vi "tcp_get_devs.vi"(8 "error in":errorcluster, 11 "TCP Network Connection in":refnum<k5>) -> (0 "error out":errorcluster, 2 "devs_info":T1[](array[typedef]), 3 "TCP Network Connection out":refnum<k5>)   [LabVIEW 2021]
uses:
  typedefs/w5500_pck.ctl
  typedefs/w5500_cmd.ctl
  typedefs/dev_full_info.ctl
  typedefs/dev_states.ctl
  typedefs/send_states.ctl
panel:
  out "dev_id":u32
  in  "dev_full_info 2":T1
  in  "devs_number":i32
  in  "w5500_pck":T4
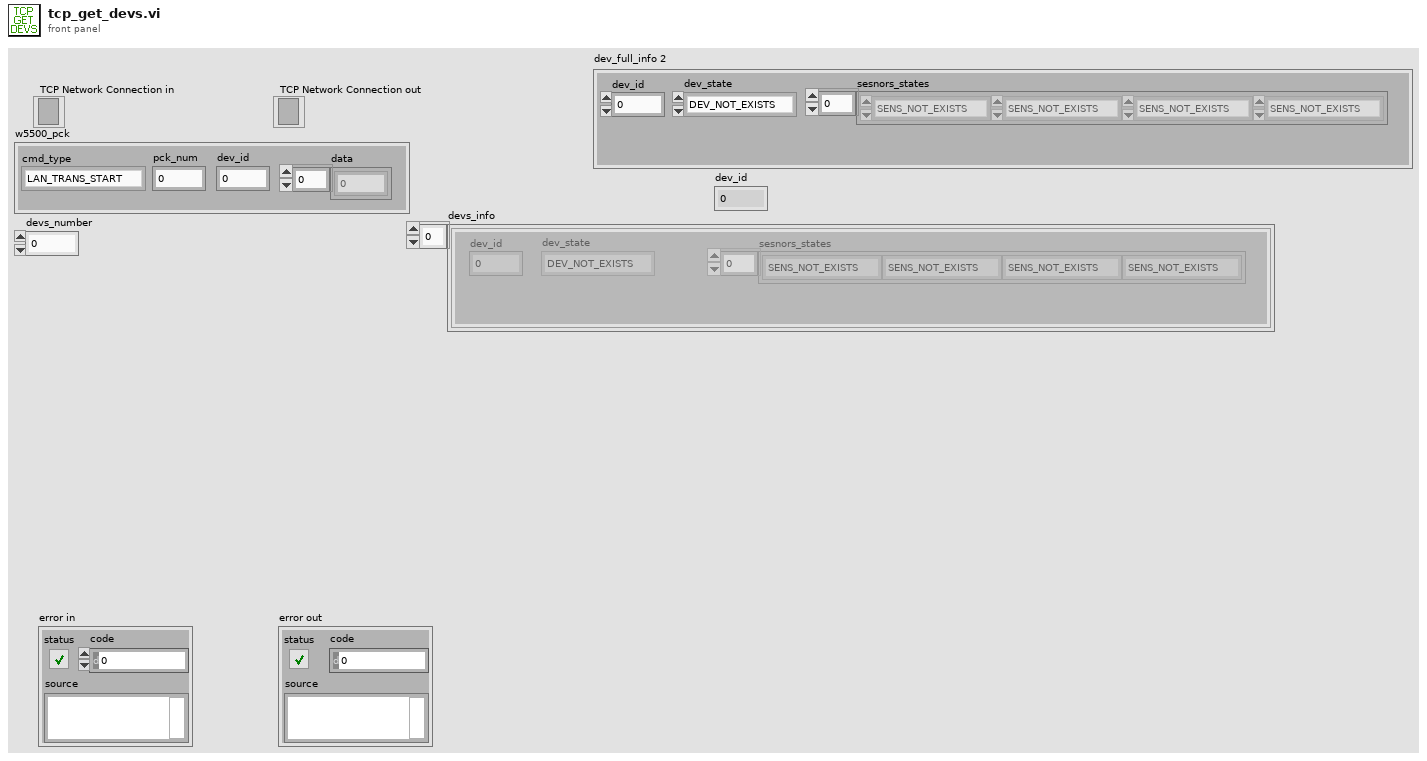
[diagram p1: front panel]
types:
  T1 = typedef "dev_full_info.ctl" = cluster{"dev_id":u32, "dev_state":T2, "sesnors_states":T3[]}
  T2 = typedef "dev_states.ctl" = enum16{"DEV_NOT_EXISTS", "DEV_EXISTS", "DEV_ERROR", "DEV_CRC_ERROR"}
  T3 = typedef "send_states.ctl" = enum16{"SENS_NOT_EXISTS", "SENS_EXISTS"}
  T4 = typedef "w5500_pck.ctl" = cluster{"cmd_type":T5, "pck_num":u32, "dev_id":u32, "data":u8[]}
  T5 = typedef "w5500_cmd.ctl" = enum32{"LAN_TRANS_START", "LAN_DATA_SZ", "LAN_CHUNK_SEND", "LAN_CHUNK_ACK", "LAN_DEVS_INFO", "LAN_DEVS_NUM", "LAN_DEVS_EXS", "LAN_DEVS_ACK", "LAN_CMD_ACK", "LAN_CMD_FIN", "LAN_SND_STAT", "LAN_REQ_STAT", "LAN_ANS_STAT", "LAN_ERR_STAT", "LAN_SETT_SET", "LAN_SETT_GET", "LAN_SETT_ACK", "LAN_SETT_ERR"}
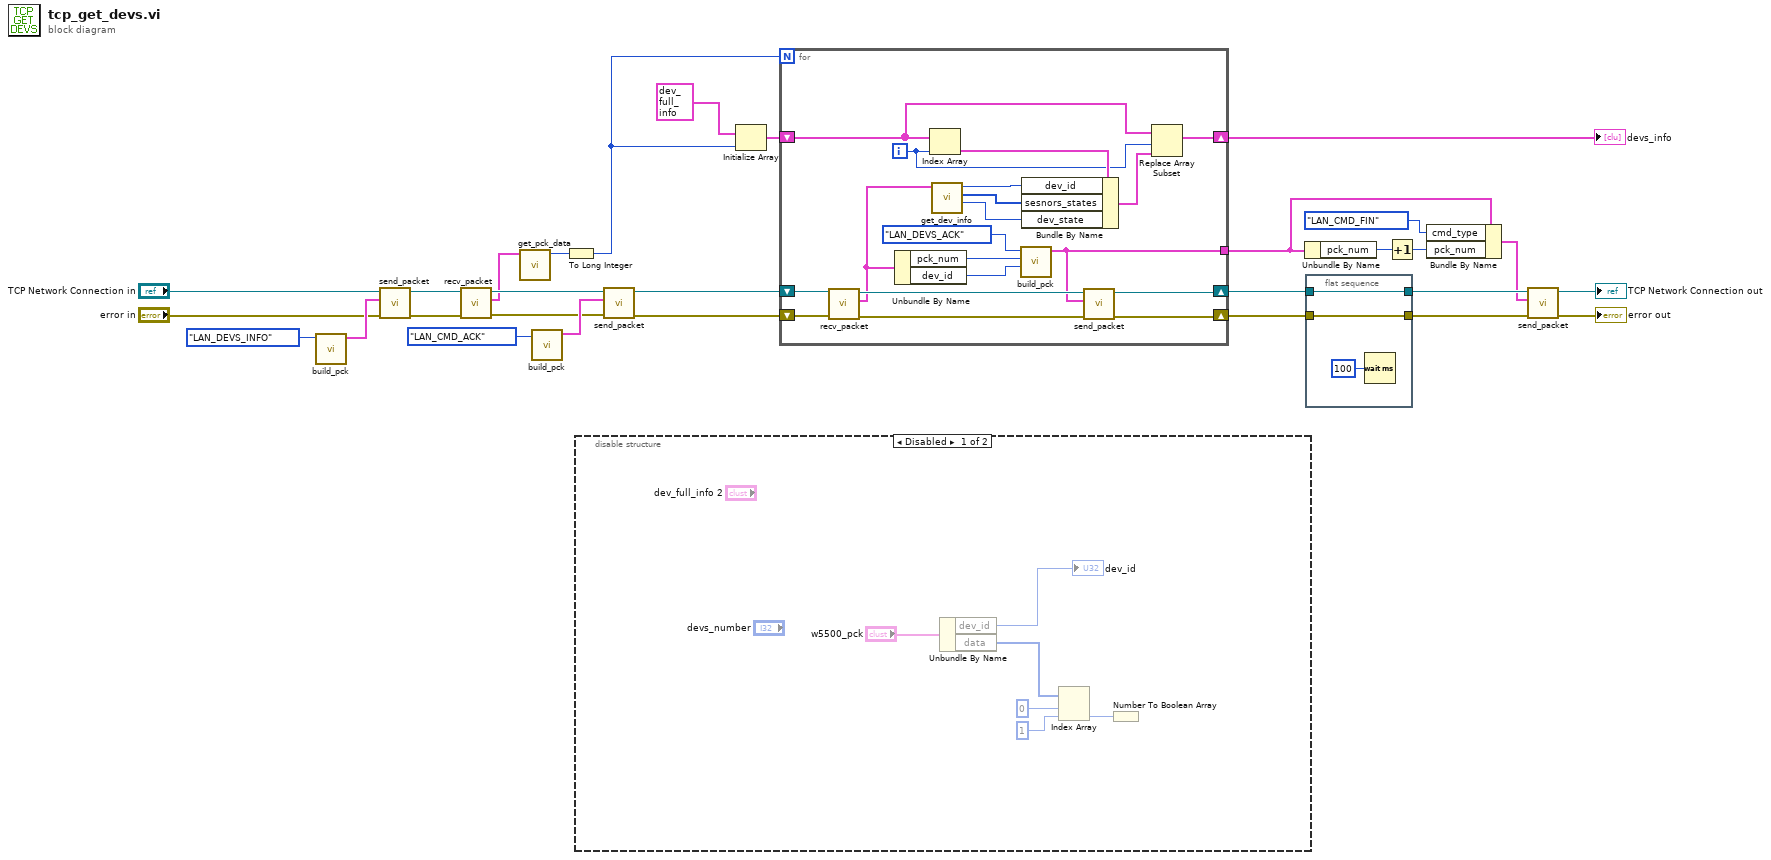
[diagram p0: block diagram]
diagram:
  n1 = call "build_pck.vi"("cmd_type"=w5500_cmd."LAN_DEVS_INFO") -> ("w5500_pck"=w25:T4)  [unwired: 10 in]
  n2 = call "send_packet.vi"("error in (no error)"="error in", "w5500_pck in"=w25, "TCP Network Connection in"="TCP Network Connection in") -> ("error out"=w22:errorcluster, "TCP Network Connection out"=w21:refnum<k5>)  [unwired: 7 in]
  n3 = call "recv_packet.vi"("error in (no error)"=w22, "TCP Network Connection in"=w21) -> ("error out"=w27:errorcluster, "w5500_pck"=w23:T4, "TCP Network Connection out"=w26:refnum<k5>)  [unwired: 7 in]
  n4 = call "get_pck_data.vi"("w5500_pck"=w23) -> ("Numeric"=w5:u32)  [unwired: 10 in]
  n5 = call "build_pck.vi"("cmd_type"=w5500_cmd."LAN_CMD_ACK") -> ("w5500_pck"=w28:T4)  [unwired: 10 in]
  n6 = To Long Integer(number=w5) -> (32bit integer=w3:i32)
  n7 = disable-structure shown="Disabled" {
    frame Disabled {
      n8 = Unbundle By Name("w5500_pck") -> ("dev_id"=→"dev_id":u32, "data"=w33:u8[])
      n9 = Index Array(array=w33, index #1=0 ("index"), index #2=1 ("index")) -> (element #2=w30:u8)  [unwired: 1 out]
      n10 = Number To Boolean Array(number=w30) -> ()  [unwired: 1 out]
    }
    frame Enabled {
    }
  }
  n11 = call "send_packet.vi"("error in (no error)"=w27, "w5500_pck in"=w28, "TCP Network Connection in"=w26) -> ("error out"=w14:errorcluster, "TCP Network Connection out"=w13:refnum<k5>)  [unwired: 7 in]
  n12 = Initialize Array(T1 {"dev_id"=0, "dev_state"=enum."DEV_NOT_EXISTS", "sesnors_states"=[enum."SENS_NOT_EXISTS", enum."SENS_NOT_EXISTS", enum."SENS_NOT_EXISTS", enum."SENS_NOT_EXISTS"]} ("dev_full_info 3"), w3) -> (w2:T1[])
  n13 = for {
    N: w3 -> [_]
    shift-right: [w49] -> w16
    shift-left: w14 -> [w53]
    shift-right: [w50] -> w15
    shift-left: w13 -> [w54]
    tunnel: [w45] -> w10
    shift-right: [w36] -> w1
    shift-left: w2 -> [w39]
    i -> [w38]
    n14 = call "recv_packet.vi"("error in (no error)"=w53, "TCP Network Connection in"=w54) -> ("error out"=w51:errorcluster, "w5500_pck"=w44:T4, "TCP Network Connection out"=w52:refnum<k5>)  [unwired: 7 in]
    n15 = Unbundle By Name(w44) -> ("pck_num"=w47:u32, "dev_id"=w46:u32)
    n16 = Index Array(array=w39, index=w38) -> (element=w43:T1)
    n17 = call "get_dev_info.vi"("w5500_pck"=w44) -> ("dev_state"=w40:T2, "sens_states"=w41:u8[], "dev_id"=w42:u32)  [unwired: 8 in]
    n18 = call "build_pck.vi"("dev_id"=w46, "pck_num"=w47, "cmd_type"=w5500_cmd."LAN_DEVS_ACK") -> ("w5500_pck"=w45:T4)  [unwired: 8 in]
    n19 = Bundle By Name(cluster=w43, "dev_id"=w42, "sesnors_states"=w41, "dev_state"=w40) -> (w37:T1)
    n20 = call "send_packet.vi"("error in (no error)"=w51, "w5500_pck in"=w45, "TCP Network Connection in"=w52) -> ("error out"=w49:errorcluster, "TCP Network Connection out"=w50:refnum<k5>)  [unwired: 7 in]
    n21 = Replace Array Subset(array=w39, new element=w37, index=w38) -> (w36:T1[])
  }
  "devs_info" <- w1
  n22 = Unbundle By Name(w10) -> ("pck_num"=w9:u32)
  n23 = flat-sequence {
    tunnel: w15 -> [w57]
    tunnel: [w57] -> w18
    tunnel: w16 -> [w56]
    tunnel: [w56] -> w17
    frame #0 {
      n24 = Wait (ms)(milliseconds to wait=u32 100) -> ()  [unwired: 1 out]
    }
  }
  n25 = Increment(x=w9) -> (x+1=w8:u32)
  n26 = Bundle By Name(cluster=w10, "cmd_type"=w5500_cmd."LAN_CMD_FIN", "pck_num"=w8) -> (w6:T4)
  n27 = call "send_packet.vi"("error in (no error)"=w17, "w5500_pck in"=w6, "TCP Network Connection in"=w18) -> ("error out"=→"error out":errorcluster, "TCP Network Connection out"=→"TCP Network Connection out":refnum<k5>)  [unwired: 7 in]
